vi "aft_LMS_Get_Copy_File_Path.vi"(8 "error in":errorcluster, 10 "filter name":string, 11 "destination folder":path) -> (0 "error out":errorcluster, 3 "destination path":path)   [LabVIEW 2017, in "NI_AdaptiveFilter.lvlib"]
uses:
  <vilib>/addons/Adaptive Filters/NI_AdaptiveFilter.lvlib
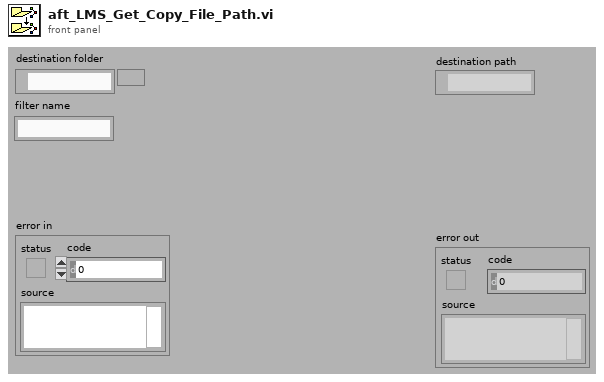
[diagram p1: front panel]
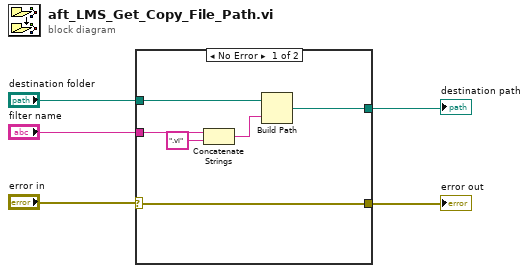
[diagram p0: block diagram]
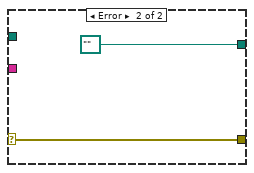
[diagram p2: hidden frame]
diagram:
  n1 = case shown="No Error" "error in" {
    selector: "error in" -> [w8 w13]
    tunnel: [w11 path ""] -> w1
    tunnel: "filter name" -> [w9 _]
    tunnel: "destination folder" -> [w10 _]
    tunnel: [w8 w13] -> w2
    frame No Error {
      n2 = Concatenate Strings(w9, ".vi") -> (w7:string)
      n3 = Build Path(base path=w10, name or relative path=w7) -> (appended path=w11:path)
    }
    frame Error {
    }
  }
  "error out" <- w2
  "destination path" <- w1
